vi "DB query example.vi"(8 "error in":errorcluster) -> (0 "error out":errorcluster, 3 "Output Array Of Clusters":T1[](array[typedef]))   [LabVIEW 2012]
uses:
  Nick's small accelerator db/nick typedef.ctl
  <vilib>/addons/database/Connection.llb/Conn Execute.vi
  <vilib>/addons/database/Recordset.llb/Rec Fetch Recordset Data (R).vi
  <vilib>/addons/database/Recordset.llb/Rec Destroy - Connection.vi
  <vilib>/addons/database/_DB Variant To Data/Database Variant To Data.xnode
  <vilib>/addons/database/NI_Database_API.lvlib
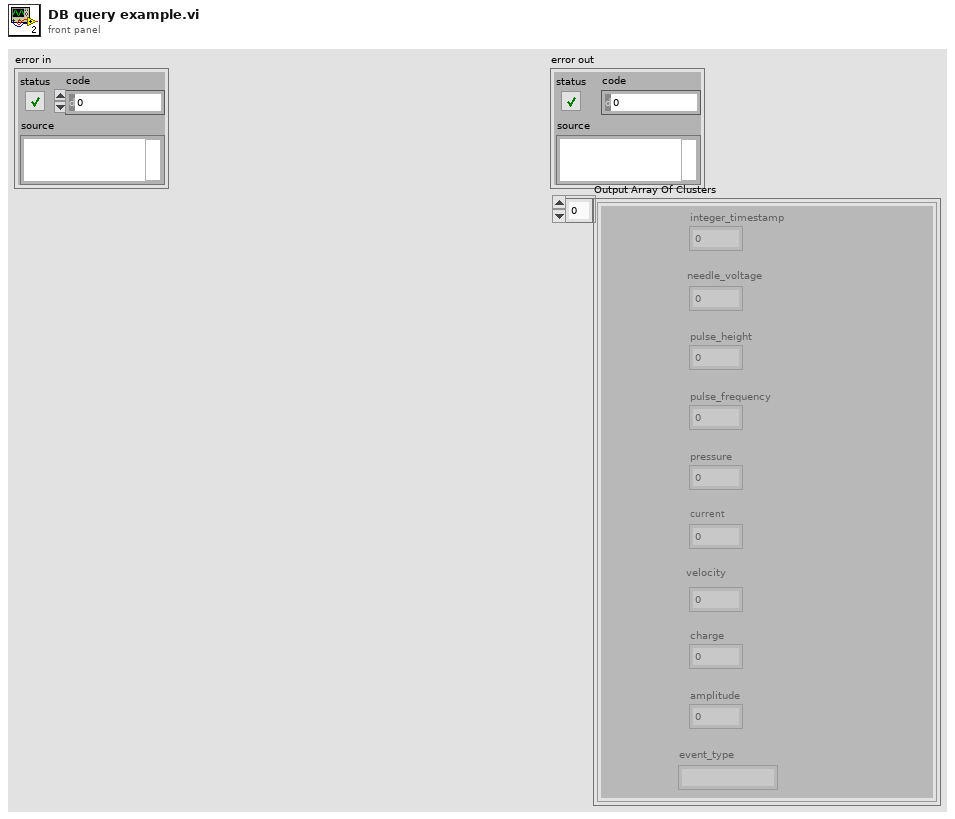
[diagram p1: front panel]
types:
  T1 = typedef "nick typedef.ctl" = cluster{"integer_timestamp":i64, "needle_voltage":dbl, "pulse_height":dbl, "pulse_frequency":dbl, "pressure":dbl, "current":dbl, "velocity":dbl, "charge":dbl, "amplitude":dbl, "event_type":string}
  T2 = typedef "NI_Database_API.lvlib/Conn ObjectReference.ctl" = refnum<k1>
  T3 = typedef "NI_Database_API.lvlib/Rec ObjectReference.ctl" = refnum<k1>
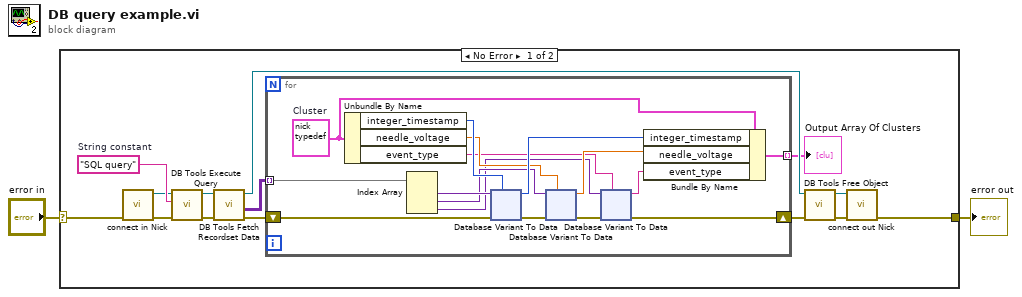
[diagram p0: block diagram]
diagram:
  n1 = case shown="No Error" "error in" {
    selector: "error in" -> [w16 w129]
    tunnel: [w15 w129] -> w1
    frame No Error {
      w13 = "SQL query"  # String constant
      n2 = call "connect in Nick.vi"("error in (no error)"=w16) -> ("error out"=w14:errorcluster, "Database Connection"=w12:T2)  [unwired: 7 in]
      n3 = call-poly <vilib>:"DB Tools Execute Query.vi"("error in (no error)"=w14, "SQL query"=w13, "connection reference"=w12) -> ("error out"=w10:errorcluster, "recordset reference"=w11:T3)  [unwired: 5 in]
      n4 = call-poly <vilib>:"DB Tools Fetch Recordset Data.vi"("error in (no error)"=w10, "recordset reference"=w11) -> ("error out"=w5:errorcluster, "recordset data"=w9:variant[][], "recordset reference out"=w8:T3)  [unwired: 3 in]
      n5 = for {
        tunnel: w9 -> [w32] mode=indexing
        shift-right: [w17] -> w4
        shift-left: w5 -> [w24]
        tunnel: [w18] -> w3 mode=indexing
        w28 = T1 {"integer_timestamp"=0, "needle_voltage"=0.0, "pulse_height"=0.0, "pulse_frequency"=0.0, "pressure"=0.0, "current"=0.0, "velocity"=0.0, "charge"=0.0, "amplitude"=0.0, "event_type"=""}  # Cluster
        n6 = Unbundle By Name(w28) -> ("integer_timestamp"=w30:i64, "needle_voltage"=w27:dbl, "event_type"=w21:string)
        n7 = Index Array(array=w32) -> (element #1=w31:variant, element #2=w25:variant, element #3=w23:variant)  [unwired: 3 in]
        n8 = xnode "Database Variant To Data"("database variant"=w31, "error in (no error)"=w24, "type"=w30) -> ("data"=w29:i64, "error out"=w20:errorcluster)
        n9 = xnode "Database Variant To Data"("database variant"=w25, "error in (no error)"=w20, "type"=w27) -> ("data"=w26:dbl, "error out"=w19:errorcluster)
        n10 = xnode "Database Variant To Data"("database variant"=w23, "error in (no error)"=w19, "type"=w21) -> ("data"=w22:string, "error out"=w17:errorcluster)
        n11 = Bundle By Name(cluster=w28, "integer_timestamp"=w29, "needle_voltage"=w26, "event_type"=w22) -> (w18:T1)
      }
      "Output Array Of Clusters" <- w3
      n12 = call-poly <vilib>:"DB Tools Free Object.vi"("error in (no error)"=w4, "recordset reference"=w8) -> ("error out"=w6:errorcluster, "connection reference"=w7:T2)  [unwired: 8 in]
      n13 = call "connect out Nick.vi"("error in (no error)"=w6, "connection reference"=w7) -> ("error out"=w15:errorcluster)  [unwired: 9 in]
    }
    frame Error {
    }
  }
  "error out" <- w1
